vi "run-vi-analyzer.vi"() -> (0 "error out":errorcluster)   [LabVIEW 2014, in "lv-cli-steps.lvlib"]
uses:
  lv-cli-steps.lvlib
  <vilib>/Utility/error.llb/DialogType.ctl
  <vilib>/Wiresmith Technology/LabVIEW CLI/CLI Class/CLI.lvclass
  <vilib>/addons/analyzer/NI_VIAnalyzerTKVIs.lvlib
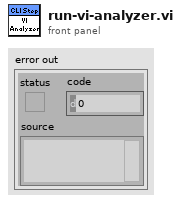
[diagram p1: front panel]
types:
  T1 = typedef "VIAnCtl Results.ctl" = cluster{"Test Name":string, "Results Data":T2[], "Status":T3, "Exceed Max Fails?":bool}
  T2 = typedef "VIAnCtl ResultsData (index).ctl" = cluster{"Result Message":string, "Ref Index":i32}
  T3 = typedef "VIAnCtl ResultStatus.ctl" = enum16{"Pass", "Fail", "Skipped", "VI not loadable", "Test not loadable", "Test not runnable", "Test error out"}
  T4 = typedef "VIAnRes Parsed Results Data (by VI).ctl" = cluster{"VI Path":path, "Pass":cluster{"row":i32, "column":i32}[], "Fail":cluster{"row":i32, "column":i32}[], "Skipped":cluster{"row":i32, "column":i32}[], "VI not loadable":cluster{"row":i32, "column":i32}[], "Test not loadable":cluster{"row":i32, "column":i32}[], "Test not runnable":cluster{"row":i32, "column":i32}[], "Test error out":cluster{"row":i32, "column":i32}[]}
  T5 = typedef "VIAnRes Parsed Results Data (by Test).ctl" = cluster{"Test Name":string, "Pass":cluster{"VI Path":path, "index":cluster{"row":i32, "column":i32}}[], "Fail":cluster{"VI Path":path, "index":cluster{"row":i32, "column":i32}}[], "Skipped":cluster{"VI Path":path, "index":cluster{"row":i32, "column":i32}}[]}
  T6 = typedef "VIAnCtl Test Config Data.ctl" = cluster{"Test Name":string, "Config Ref":refnum<vi>, "Ref Valid?":bool, "Test Ranking":T7, "Max Failures":u32, "Test Path":path, "Control Values":T8[], "Selected?":bool}
  T7 = typedef "VIAnCtl TestRanking.ctl" = u16
  T8 = typedef "VIAnCtl Config Control Value.ctl" = cluster{"Control Name":string, "Control Value":variant}
  T9 = cluster{"Raw Results":T1[][], "Parsed Results Data (by VI)":T4[], "Parsed Results Data (by Test)":T5[], "Summary Statistics":cluster{"Passed Tests":i32, "Failed Tests":i32, "Skipped Tests":i32, "VIs not loadable":i32, "Tests not loadable":i32, "Tests not runnable":i32, "Test error out":i32, "Start Time":u32, "Total Time (s)":dbl}, "Test Config Data":T6[]}
  T10 = typedef "DialogType.ctl" = u16
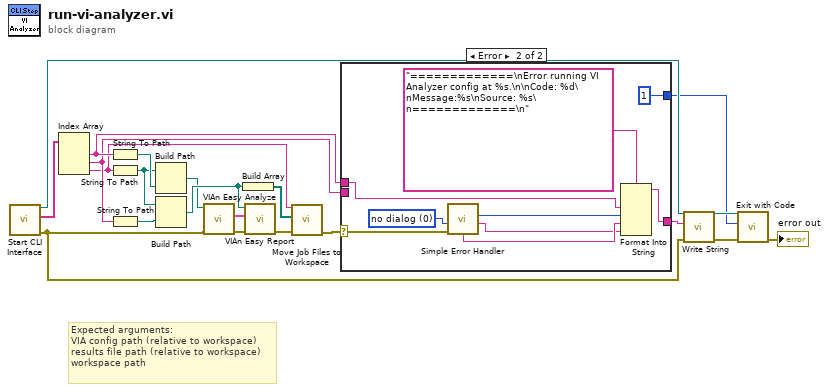
[diagram p0: block diagram]
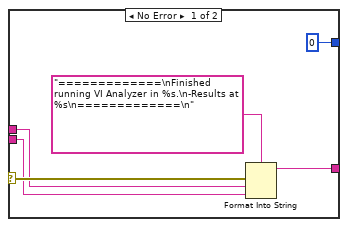
[diagram p2: hidden frame]
diagram:
  # "Expected arguments:\nVIA config path (relative to workspace)\nresults file path (relative to workspace)\nworkspace path"
  n1 = call <vilib>:"Start CLI Interface.vi"() -> ("error out"=w1:errorcluster, "Custom Parameters"=w21:string[], "CLI out"=w17:refnum<class "CLI.lvclass">)  [unwired: 9 in]
  n2 = Index Array(array=w21) -> (element #1=w20:string, element #2=w19:string, element #3=w9:string)  [unwired: 3 in]
  n3 = String To Path(string=w20) -> (path=w13:path)
  n4 = String To Path(string=w9) -> (path=w12:path)
  n5 = String To Path(string=w19) -> (path=w11:path)
  n6 = Build Path(base path=w12, name or relative path=w13) -> (appended path=w2:path)
  n7 = Build Path(base path=w12, name or relative path=w11) -> (appended path=w3:path)
  n8 = call <vilib>:"VIAn Easy Analyze.vi"("error in (no error)"=w1, "Analysis Target"=w2) -> ("error out"=w6:errorcluster, "Analysis Results"=w5:T9)  [unwired: 8 in]
  n9 = Build Array(w3) -> (w10:path[])
  n10 = call <vilib>:"VIAn Easy Report.vi"("error in (no error)"=w6, "Analysis Results"=w5, "Report Save Path"=w3) -> ("error out"=w4:errorcluster)  [unwired: 8 in]
  n11 = call "Move Job Files to Workspace.vi"("error in (no error)"=w4, "Generated Files"=w10, "Workspace Path"=w9) -> ("error out"=w8:errorcluster)  [unwired: 8 in]
  n12 = case shown="Error" w8 {
    selector: w8 -> [w26 w35]
    tunnel: w20 -> [w25 w31]
    tunnel: w19 -> [w24 _]
    tunnel: [w23 w36] -> w18
    tunnel: [0 ("Exit Code (0)") 1 ("Exit Code (0)")] -> w14
    frame No Error {
      n13 = Format Into String(format string="=============\nFinished running VI Analyzer in %s.\n-Results at %s\n=============\n", error in=w26, w25, w24) -> (resulting string=w23:string)  [unwired: 1 in, 1 out]
    }
    frame Error {
      w34 = T10 0 items=["no dialog", "OK message", "continue or stop message", "OK message + warnings", "continue/stop + warnings"] ("type of dialog (OK msg:1)")
      n14 = call <vilib>:"Simple Error Handler.vi"("type of dialog (OK msg:1)"=w34, "error in (no error)"=w35) -> ("code out"=w28:i32, "source out"=w29:string, "message"=w30:string)  [unwired: 3 in, 2 out]
      n15 = Format Into String(format string="=============\nError running VI Analyzer config at %s.\n\nCode: %d\nMessage:%s\nSource: %s\n=============\n", w31, w28, w30, w29) -> (resulting string=w36:string)  [unwired: 2 in, 1 out]
    }
  }
  n16 = call <vilib>:"Write String.vi"("error in (no error)"=w1, "Text to Write"=w18, "CLI in"=w17) -> ("error out"=w16:errorcluster, "CLI out"=w15:refnum<class "CLI.lvclass">)  [unwired: 7 in]
  n17 = call <vilib>:"Exit with Code.vi"("error in (no error)"=w16, "Exit Code (0)"=w14, "CLI in"=w15) -> ("error out"=→"error out":errorcluster)  [unwired: 8 in]
